vi "2 D Array infinity table generate.vi"() -> ()   [LabVIEW 2015]
panel:
  in  "x":dbl
  out "Array":i32[][](array[numeric])
  # "2 D Array infinity tabale generate"
  # "Pardeep Kumar"
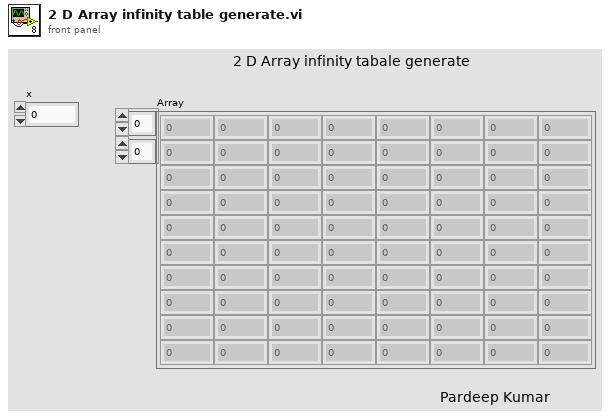
[diagram p1: front panel]
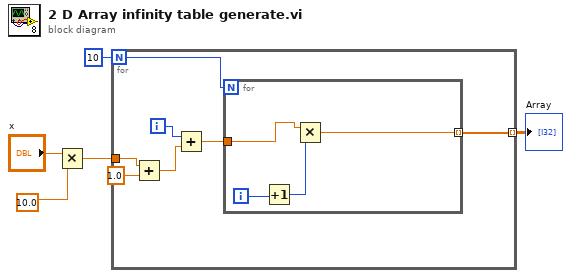
[diagram p0: block diagram]
diagram:
  n1 = Multiply(x="x", y=10.0) -> (x*y=w1:dbl)
  n2 = for {
    N: 10 -> [w12]
    tunnel: [w9] -> w4 mode=indexing
    tunnel: w1 -> [w7]
    i -> [w11]
    n3 = Add(x=w7, y=1.0) -> (x+y=w8:dbl)
    n4 = Add(x=w11, y=w8) -> (x+y=w10:dbl)
    n5 = for {
      N: w12 -> [_]
      tunnel: w10 -> [w16]
      tunnel: [w15] -> w9 mode=indexing
      i -> [w14]
      n6 = Increment(x=w14) -> (x+1=w13:i32)
      n7 = Multiply(x=w16, y=w13) -> (x*y=w15:dbl)
    }
  }
  "Array" <- w4
